vi "pwm_rpmPIP.vi"(8 "error in (no error)":errorcluster) -> (0 "error out":errorcluster, 3 "PWM_RPM":string)   [LabVIEW 2018]
uses:
  Global_1259.vi
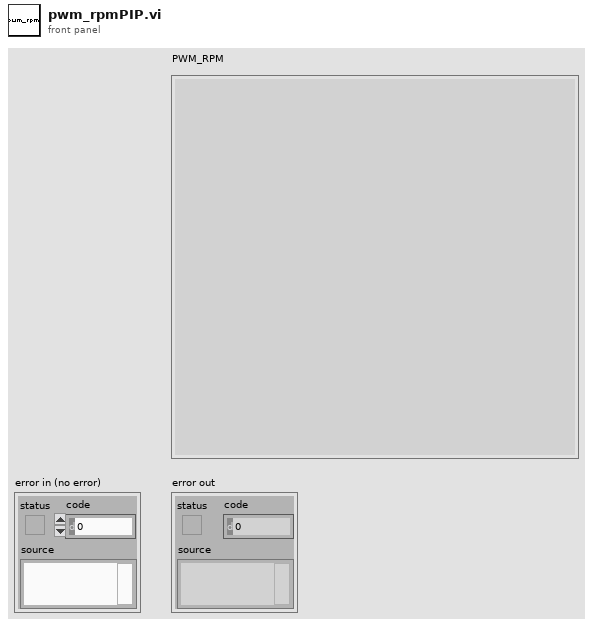
[diagram p1: front panel]
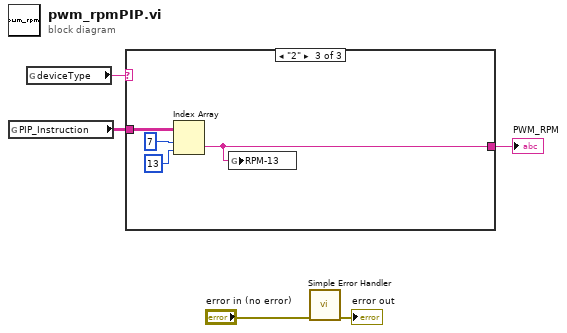
[diagram p0: block diagram]
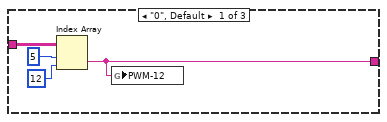
[diagram p2: hidden frame]
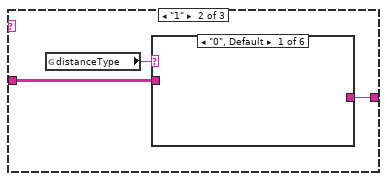
[diagram p3: hidden frame]
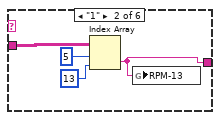
[diagram p4: hidden frame]
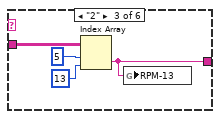
[diagram p5: hidden frame]
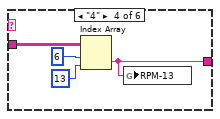
[diagram p6: hidden frame]
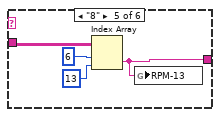
[diagram p7: hidden frame]
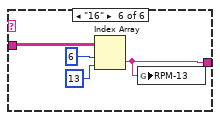
[diagram p8: hidden frame]
diagram:
  n1 = global read "Global_1259.vi" "PIP_Instruction"() -> (w1:string[][])
  n2 = global read "Global_1259.vi" "deviceType"() -> (w5:string)
  n3 = case shown="\"2\"" w5 {
    tunnel: w1 -> [w9 w12 w36]
    tunnel: [w6 w11 w33] -> w4
    frame "0", Default {
      n4 = Index Array(array=w9, index (row)=5, index (col)=12 ("disabled index (col)")) -> (element=w6:string)
      n5 = global write "Global_1259.vi" "PWM-12"(w6) -> ()
    }
    frame "1" {
      n6 = global read "Global_1259.vi" "distanceType"() -> (w10:string)
      n7 = case shown="\"0\", Default" w10 {
        tunnel: w12 -> [_ w14 w18 w22 w26 w30]
        tunnel: [_ w13 w17 w21 w25 w29] -> w11
        frame "0", Default {
        }
        frame "1" {
          n8 = Index Array(array=w14, index (row)=5, index (col)=13 ("disabled index (col)")) -> (element=w13:string)
          n9 = global write "Global_1259.vi" "RPM-13"(w13) -> ()
        }
        frame "2" {
          n10 = Index Array(array=w18, index (row)=5, index (col)=13 ("disabled index (col)")) -> (element=w17:string)
          n11 = global write "Global_1259.vi" "RPM-13"(w17) -> ()
        }
        frame "4" {
          n12 = Index Array(array=w22, index (row)=6, index (col)=13 ("disabled index (col)")) -> (element=w21:string)
          n13 = global write "Global_1259.vi" "RPM-13"(w21) -> ()
        }
        frame "8" {
          n14 = Index Array(array=w26, index (row)=6, index (col)=13 ("disabled index (col)")) -> (element=w25:string)
          n15 = global write "Global_1259.vi" "RPM-13"(w25) -> ()
        }
        frame "16" {
          n16 = Index Array(array=w30, index (row)=6, index (col)=13 ("disabled index (col)")) -> (element=w29:string)
          n17 = global write "Global_1259.vi" "RPM-13"(w29) -> ()
        }
      }
    }
    frame "2" {
      n18 = Index Array(array=w36, index (row)=7, index (col)=13 ("disabled index (col)")) -> (element=w33:string)
      n19 = global write "Global_1259.vi" "RPM-13"(w33) -> ()
    }
  }
  "PWM_RPM" <- w4
  n20 = call <vilib>:"Simple Error Handler.vi"("error in (no error)"="error in (no error)") -> ("error out"=→"error out":errorcluster)  [unwired: 4 in, 4 out]
